vi "ParametersUpdated.vi"(8 "error in (no error)":errorcluster, 10 "Spectro Parameters":T1, 11 "SpectroscopyUI in":refnum<class "SpectroscopyUI.lvclass">) -> (0 "error out":errorcluster, 3 "SpectroscopyUI out":refnum<class "SpectroscopyUI.lvclass">)   [LabVIEW 2023, in "SpectroscopyUI.lvlib" / "SpectroscopyUI.lvclass"]
uses:
  SpectroscopyUI.lvclass
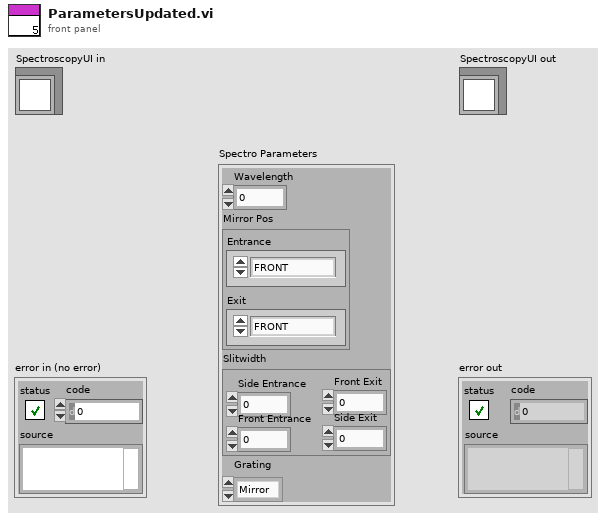
[diagram p1: front panel]
types:
  T1 = cluster{"Wavelength":dbl, "Mirror Pos":cluster{"Entrance":enum16{"FRONT", "SIDE"}, "Exit":enum16{"FRONT", "SIDE"}}, "Slitwidth":cluster{"Side Entrance":u16, "Front Entrance":u16, "Front Exit":u16, "Side Exit":u16}, "Grating":enum16{"Mirror", "1200 g/mm", "1800 g/mm"}}
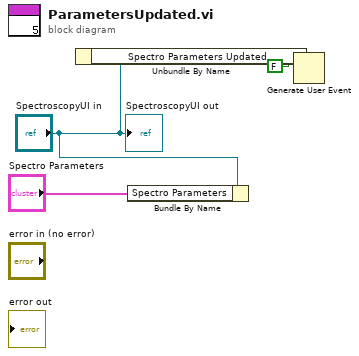
[diagram p0: block diagram]
diagram:
  n1 = Unbundle By Name("SpectroscopyUI in") -> ("Spectro Parameters Updated"=w2:refnum<user-event>)
  n2 = Bundle By Name(cluster="SpectroscopyUI in", "Spectro Parameters"="Spectro Parameters") -> ()  [unwired: 1 out]
  n3 = Generate User Event(user event=w2, event data cluster=FALSE ("event data")) -> ()  [unwired: 2 in, 2 out]
  "SpectroscopyUI out" <- "SpectroscopyUI in"
